vi "Read col.vi"(8 "error in (no error)":errorcluster, 11 "BoardField in":refnum<class "BoardField.lvclass">) -> (0 "error out":errorcluster, 2 "col":u8, 3 "BoardField out":refnum<class "BoardField.lvclass">)   [LabVIEW 2017, in "BoardField.lvclass"]
uses:
  BoardField.lvclass
  BoardField.lvclass/BoardField.ctl
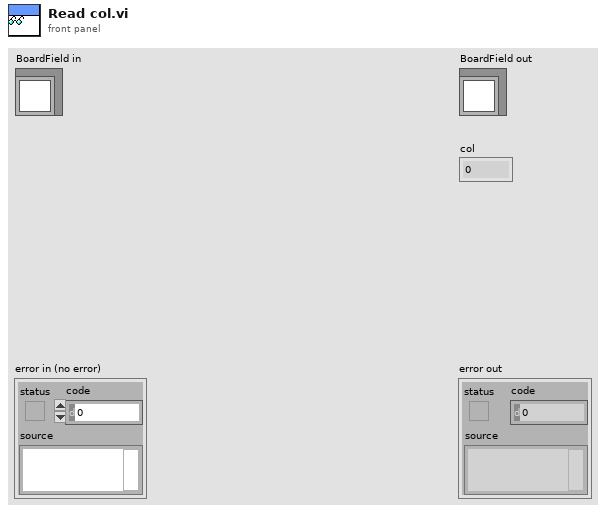
[diagram p1: front panel]
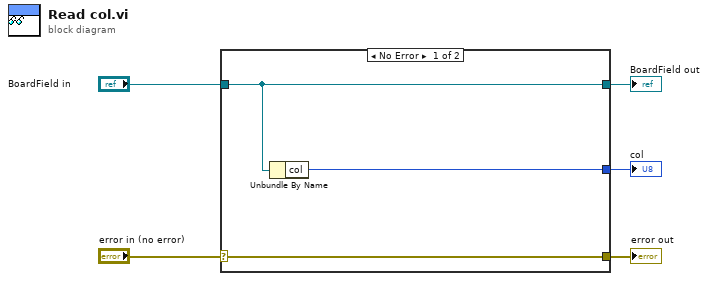
[diagram p0: block diagram]
diagram:
  n1 = case shown="No Error" "error in (no error)" {
    selector: "error in (no error)" -> [w8 w9]
    tunnel: [w8 w9] -> w4
    tunnel: [w7 w10] -> w2
    tunnel: "BoardField in" -> [w7 w10]
    tunnel: [w6 _] -> w1
    frame No Error {
      n2 = Unbundle By Name(w7) -> ("col"=w6:u8)
    }
    frame Error {
    }
  }
  "error out" <- w4
  "BoardField out" <- w2
  "col" <- w1
